vi "Calibration.vi"(8 "error in (no error)":errorcluster, 9 "ADC possitions":dbl[](array[numeric]), 10 "ADC Distance (mm)":dbl, 11 "TCP Network Connection in":refnum<k5>) -> (0 "error out":errorcluster, 1 "clabration running":bool, 2 "Possition index":i32, 3 "TCP Network Connection out":refnum<k5>)   [LabVIEW 2019]
panel:
  out "Cup Position":T1(ring)
  out "sorted array":dbl[](array[numeric])
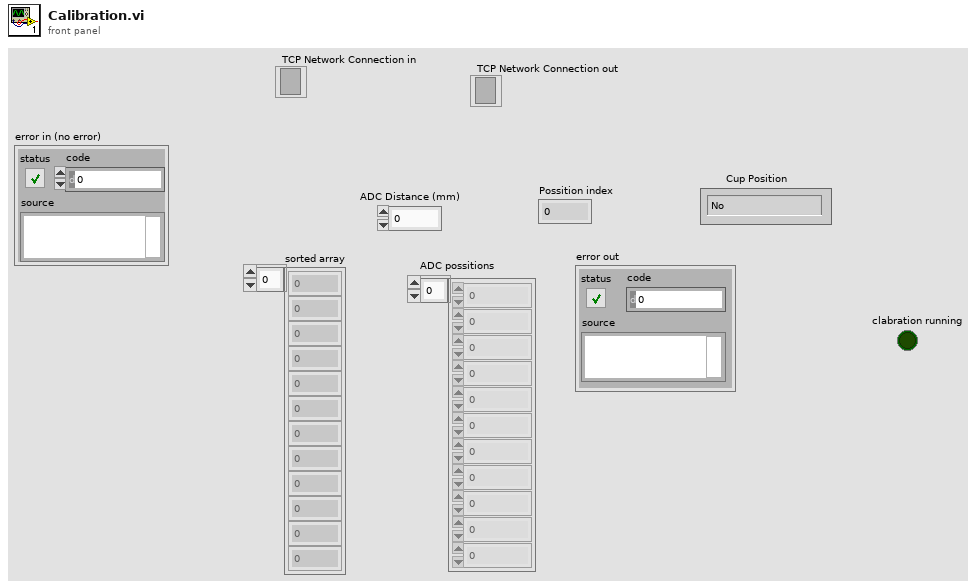
[diagram p1: front panel]
types:
  T1 = enum16{"No", "Home", "Anneal", "Bottom Cup", "Middle Cup", "Top Cup"}
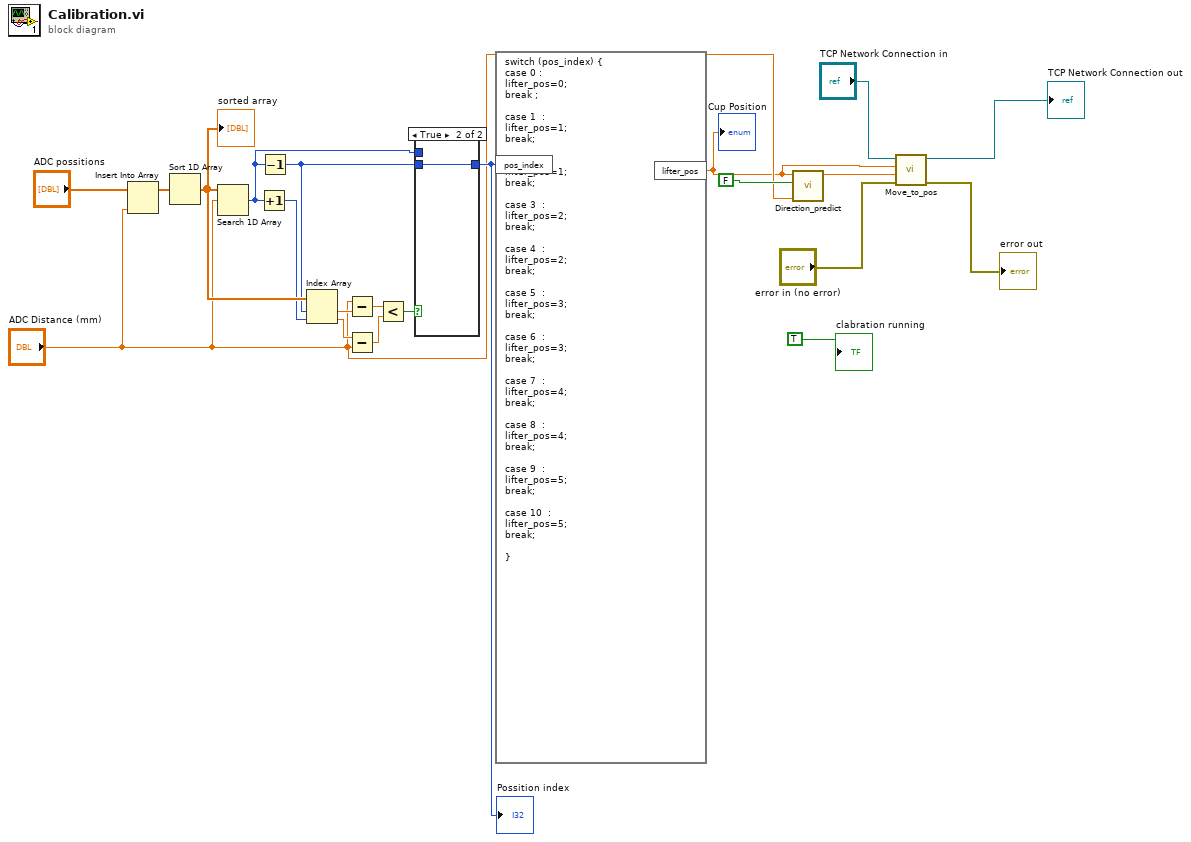
[diagram p0: block diagram]
diagram:
  n1 = Insert Into Array(array="ADC possitions", new element="ADC Distance (mm)") -> (w21:dbl[])  [unwired: 1 in]
  n2 = Sort 1D Array(array=w21) -> (sorted array=w20:dbl[])
  "sorted array" <- w20
  n3 = Search 1D Array(1D array=w20, element="ADC Distance (mm)") -> (index of element=w11:i32)  [unwired: 1 in]
  n4 = Increment(x=w11) -> (x+1=w12:i32)
  n5 = Decrement(x=w11) -> (x-1=w13:i32)
  n6 = Index Array(array=w20, index #1=w13, index #2=w12) -> (element #1=w14:dbl, element #2=w15:dbl)
  n7 = Subtract(x="ADC Distance (mm)", y=w14) -> (x-y=w18:dbl)
  n8 = Subtract(x=w15, y="ADC Distance (mm)") -> (x-y=w17:dbl)
  n9 = Less?(x=w18, y=w17) -> (x < y?=w16:bool)
  n10 = case shown="True" w16 {
    tunnel: w13 -> [_ w23]
    tunnel: [w22 w23] -> w10
    tunnel: w11 -> [w22 _]
    frame False {
    }
    frame True {
    }
  }
  "Possition index" <- w10
  n11 = formula code="switch (pos_index) {\ncase 0 : \nlifter_pos=0;\nbreak ;\n\ncase 1  : \nlifter_pos=1;\nbreak;\n\ncase 2  : \nlifter_pos=1;\nbreak;\n\ncase 3  : \nlifter_pos=2;\nbreak;\n\ncase 4  : \nlifter_pos=2;\nbreak;\n\ncase 5  : \nlifter_pos=3;\nbreak;\n\ncase 6  : \nlifter_pos=3;\nbreak;\n\ncase 7  : \nlifter_pos=4;\nbreak;\n\ncase 8  : \nlifter_pos=4;\nbreak;\n\ncase 9  : \nlifter_pos=5;\nbreak;\n\ncase 10  : \nlifter_pos=5;\nbreak;\n\n}"("pos_index"=w10) -> ("lifter_pos"=w6:dbl)
  "Cup Position" <- w6
  n12 = call "Direction_predict.vi"("ADC distance"="ADC Distance (mm)", "Step status"=FALSE, "Cup Position"=w6) -> ("Direction"=w7:dbl)  [unwired: 8 in]
  n13 = call "Move_to_pos.vi"("error in (no error)"="error in (no error)", "Direction"=w7, "Cup Position"=w6, "TCP Network Connection in"="TCP Network Connection in") -> ("error out"=→"error out":errorcluster, "TCP Network Connection out"=→"TCP Network Connection out":refnum<k5>)  [unwired: 6 in]
  "clabration running" <- TRUE ("clabration running")
